vi "Read VISA resource name.vi"(8 "error in (no error)":errorcluster, 11 "Strain Digitizer in":refnum<class "Micron sm Digitizer.lvclass">) -> (0 "error out":errorcluster, 2 "VISA resource name":refnum<visa-resource-name>="TCPIP0::192.168.1.69::1852::SOCKET", 3 "Strain Digitizer out":refnum<class "Micron sm Digitizer.lvclass">)   [LabVIEW 2024]
uses:
  Micron sm Digitizer.lvclass
  Micron sm Digitizer.lvclass/Micron sm Digitizer.ctl
  D:/GitHub/NHMFL_Core/Libraries/Instruments/Micron Optics/Micron Optics Driver/Micron Optics Driver.lvclass
  D:/GitHub/NHMFL_Core/Libraries/Instruments/Spectrometer Driver/Spectrometer Driver.lvclass
  D:/GitHub/NHMFL_Core/Libraries/Instruments/Pulse Driver/Pulse Driver.lvclass
  D:/GitHub/NHMFL_Core/Libraries/Instruments/Simple VISA Reader/Simple VISA Reader Driver.lvclass
  D:/GitHub/NHMFL_Core/Libraries/Instruments/VISA Instrument/VISA Instrument.lvclass
  D:/GitHub/NHMFL_Core/Libraries/Instruments/Instrument Driver/Instrument Driver.lvclass
  D:/GitHub/NHMFL_Core/Libraries/Instruments/Strain Digitizer/Micron sm Digitizer.lvclass
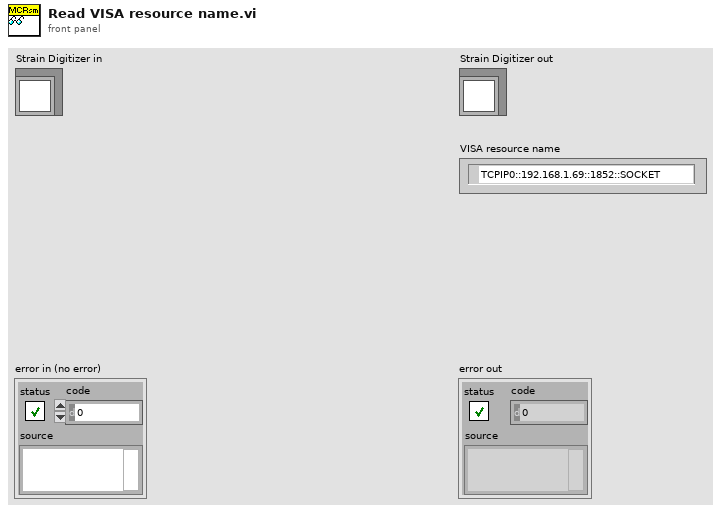
[diagram p1: front panel]
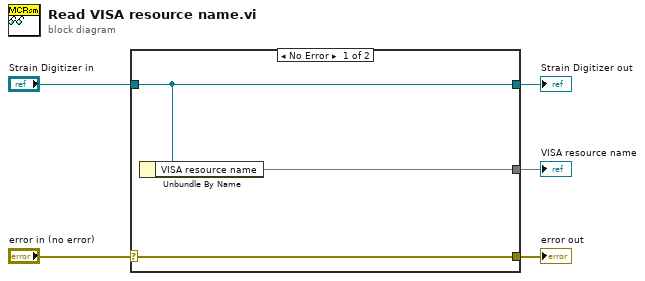
[diagram p0: block diagram]
diagram:
  n1 = case shown="No Error" "error in (no error)" {
    selector: "error in (no error)" -> [w8 w9]
    tunnel: [w8 w9] -> w4
    tunnel: [w7 w10] -> w2
    tunnel: "Strain Digitizer in" -> [w7 w10]
    tunnel: [w6 _] -> w1
    frame No Error {
      n2 = Unbundle By Name(w7) -> ("VISA resource name"=w6)
    }
    frame Error {
    }
  }
  "error out" <- w4
  "Strain Digitizer out" <- w2
  "VISA resource name" <- w1
